vi "Preset PART NUMBER validator.vi"(8 "error in (no error)":errorcluster, 10 "PART number":string, 11 "VISA resource in":refnum<visa-resource-name>) -> (0 "error out":errorcluster, 3 "VISA resource out":refnum<visa-resource-name>)   [LabVIEW 2025, in "Chroma 19052.lvlib"]
uses:
  <instrlib>/Chroma 19052/Chroma 19052.lvlib
  <instrlib>/Chroma 19052/Public/Utility/Type Def/Preset Number States--enum.ctl
panel:
  # "Set PART number  with validation"
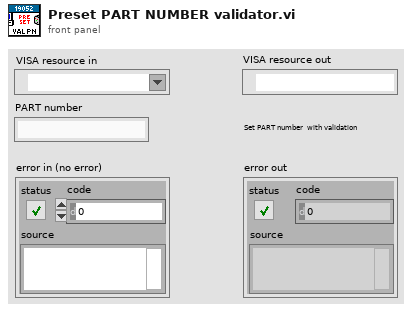
[diagram p1: front panel]
types:
  T1 = typedef "Chroma 19052.lvlib/Preset Number States--enum.ctl" = enum16{"Initialize", "Check <=UL", "Check >=LL", "Truncate string", "Send command", "Shutdown"}
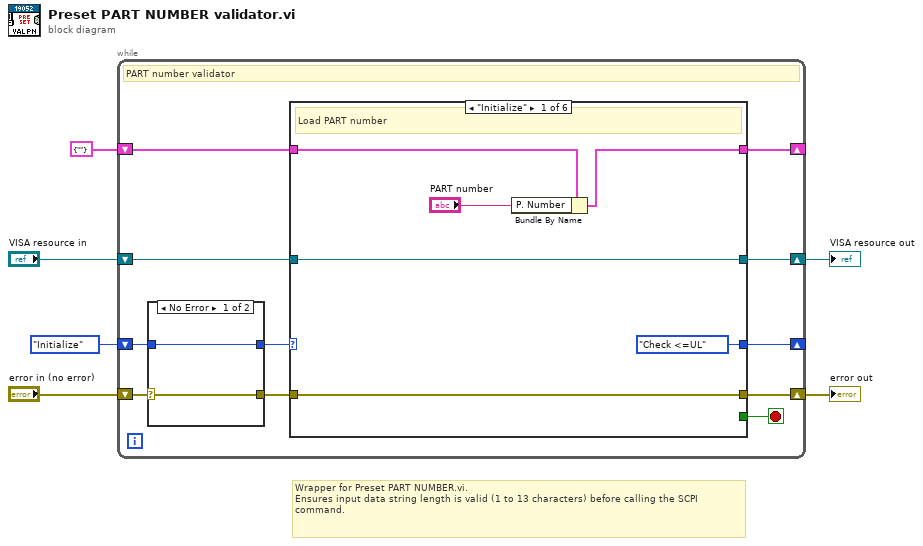
[diagram p0: block diagram]
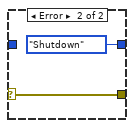
[diagram p2: hidden frame]
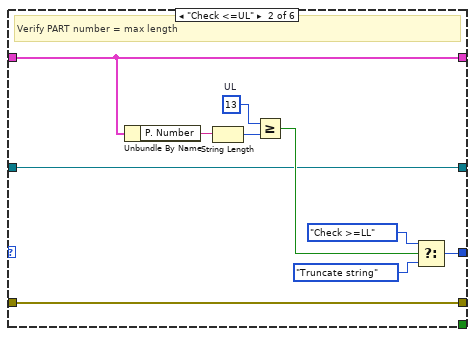
[diagram p3: hidden frame]
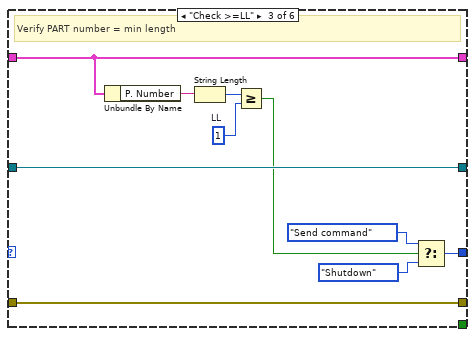
[diagram p4: hidden frame]
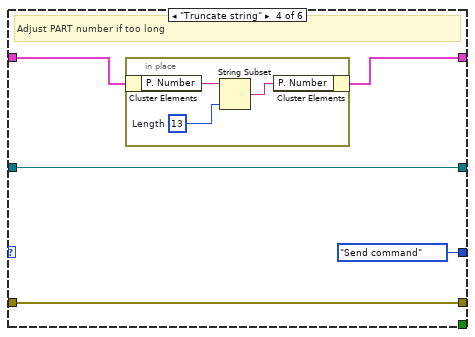
[diagram p5: hidden frame]
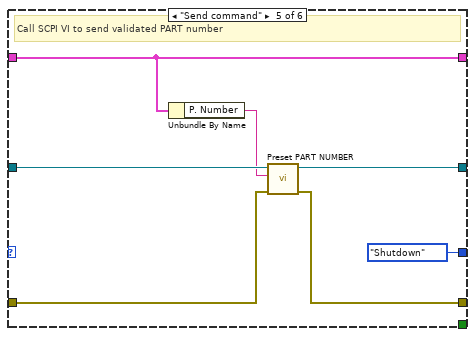
[diagram p6: hidden frame]
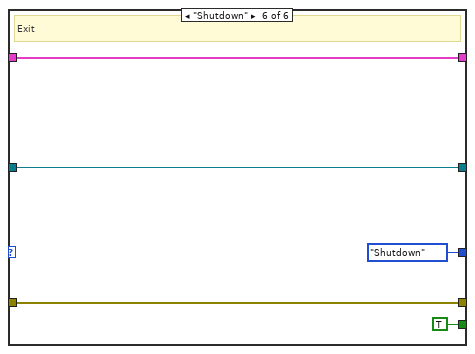
[diagram p7: hidden frame]
diagram:
  # "Wrapper for Preset PART NUMBER.vi.\nEnsures input data string length is valid (1 to 13 characters) before calling the SCPI command."
  n1 = while {
    shift-right: [w15] -> _
    shift-left: Preset_Number_States--enum."Initialize" -> [w14]
    shift-right: [w10] -> w3
    shift-left: "VISA resource in" -> [w13]
    shift-right: [w8] -> _
    shift-left: cluster{"P. Number":string} {"P. Number"=""} -> [w7]
    shift-right: [w11] -> w4
    shift-left: "error in (no error)" -> [w16]
    stop <- w9 stop-if-true
    # "PART number validator"
    n2 = case shown="No Error" w16 {
      selector: w16 -> [w19 w21]
      tunnel: [w19 w21] -> w12
      tunnel: [w18 Preset_Number_States--enum."Shutdown"] -> w17
      tunnel: w14 -> [w18 _]
      frame No Error {
      }
      frame Error {
      }
    }
    n3 = case shown="\"Initialize\"" w17 {
      tunnel: [Preset_Number_States--enum."Check <=UL" w34 w43 Preset_Number_States--enum."Send command" Preset_Number_States--enum."Shutdown" Preset_Number_States--enum."Shutdown"] -> w15
      tunnel: w13 -> [w26 w33 w47 w52 w60 w67]
      tunnel: w12 -> [w27 w32 w46 w51 w58 w66]
      tunnel: [w27 w32 w46 w51 w57 w66] -> w11
      tunnel: [w26 w33 w47 w52 w59 w67] -> w10
      tunnel: [_ _ _ _ _ TRUE] -> w9
      tunnel: w7 -> [w25 w31 w40 w49 w61 w63]
      tunnel: [w24 w31 w40 w48 w61 w63] -> w8
      frame "Initialize" {
        # "Load PART number"
        n4 = Bundle By Name(cluster=w25, "P. Number"="PART number") -> (w24:cluster{"P. Number":string})
      }
      frame "Check <=UL" {
        w37 = 13  # UL
        # "Verify PART number = max length"
        n5 = Unbundle By Name(w31) -> ("P. Number"=w30:string)
        n6 = String Length(string=w30) -> (length=w36:i32)
        n7 = Greater Or Equal?(x=w37, y=w36) -> (x >= y?=w35:bool)
        n8 = Select(t=Preset_Number_States--enum."Check >=LL", s=w35, f=Preset_Number_States--enum."Truncate string") -> (s? t:f=w34:T1)
      }
      frame "Check >=LL" {
        w44 = 1  # LL
        # "Verify PART number = min length"
        n9 = Unbundle By Name(w40) -> ("P. Number"=w39:string)
        n10 = String Length(string=w39) -> (length=w45:i32)
        n11 = Greater Or Equal?(x=w45, y=w44) -> (x >= y?=w42:bool)
        n12 = Select(t=Preset_Number_States--enum."Send command", s=w42, f=Preset_Number_States--enum."Shutdown") -> (s? t:f=w43:T1)
      }
      frame "Truncate string" {
        # "Adjust PART number if too long"
        n13 = in-place "In Place Element Structure" {
          w55 = 13  # Length
          n14 = in-place-cluster #1 ("Unbundle / Bundle Elements")(w49) -> ("P. Number"=w54:string)
          n15 = String Subset(string=w54, length (rest)=w55) -> (substring=w53:string)  [unwired: 1 in]
          n16 = in-place-cluster #1 ("Unbundle / Bundle Elements")("P. Number"=w53) -> (w48:cluster{"P. Number":string})
        }
      }
      frame "Send command" {
        # "Call SCPI VI to send validated PART number"
        n17 = Unbundle By Name(w61) -> ("P. Number"=w56:string)
        n18 = call <instrlib>:"Preset PART NUMBER.vi"("error in (no error)"=w58, "PART number"=w56, "VISA Refnum in"=w60) -> ("error out"=w57:errorcluster, "VISA Refnum out"=w59:refnum<visa-resource-name>)  [unwired: 7 in]
      }
      frame "Shutdown" {
        # "Exit"
      }
    }
  }
  "error out" <- w4
  "VISA resource out" <- w3
